vi "Execute Operation.vi"(6 "Operation":T1(ring), 8 "error in (no error)":errorcluster, 9 "Op 2":dbl, 10 "Op 1":dbl, 11 "Controller in":refnum<class "Controller.lvclass">) -> (0 "error out":errorcluster, 3 "Controller out":refnum<class "Controller.lvclass">)   [LabVIEW 2013, in "Controller.lvlib" / "Controller.lvclass"]
uses:
  Controller.lvclass
  Controller.lvclass/Controller.ctl
  Calculate/Calculate Messages/Calculate Msg/Calculate Msg.lvclass/Calculate Msg.ctl
  <vilib>/ActorFramework/Message Enqueuer/Message Enqueuer.lvclass/Message Enqueuer.ctl
  <vilib>/ActorFramework/Message Enqueuer/Enqueue.vi
  <vilib>/ActorFramework/Message Priority Queue/Priority Enqueue.vi
  Calculate/Calculate Messages/Calculate Msg/Calculate Msg.lvclass
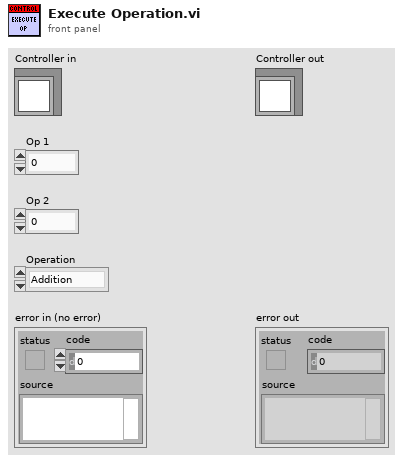
[diagram p1: front panel]
types:
  T1 = enum16{"Addition", "Subtraction", "Multiply", "Divide"}
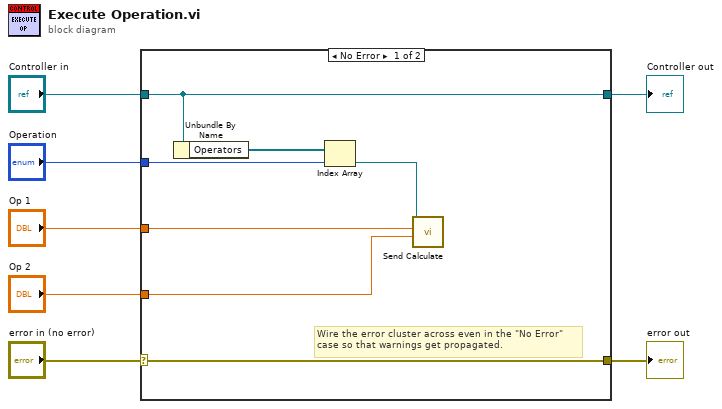
[diagram p0: block diagram]
diagram:
  n1 = case shown="No Error" "error in (no error)" {
    selector: "error in (no error)" -> [w14 w16]
    tunnel: [w14 w16] -> w6
    tunnel: [w13 w15] -> w4
    tunnel: "Controller in" -> [w13 w15]
    tunnel: "Operation" -> [w11 _]
    tunnel: "Op 1" -> [w9 _]
    tunnel: "Op 2" -> [w8 _]
    frame No Error {
      # "Wire the error cluster across even in the \"No Error\"\ncase so that warnings get propagated."
      n2 = Unbundle By Name(w13) -> ("Operators"=w12:refnum<class "Message Enqueuer.lvclass">[])
      n3 = Index Array(array=w12, index=w11) -> (element=w10:refnum<class "Message Enqueuer.lvclass">)
      n4 = call "Send Calculate.vi"("Operand 2"=w8, "Operand 1"=w9, "Message Enqueuer"=w10) -> ()  [unwired: 7 in, 2 out]
    }
    frame Error {
    }
  }
  "error out" <- w6
  "Controller out" <- w4
